vi "h.DETECTION.GetAllChannelDetectionSettingIds.vi"(8 "error in":errorcluster, 11 "Connection ID":refnum<k5>) -> (0 "error out":errorcluster, 2 "Detection Settings IDs":u8[](array[numeric]), 3 "Connection ID out":refnum<k5>)   [LabVIEW 2016, in "h.Library.lvlib"]
uses:
  h.Library.lvlib
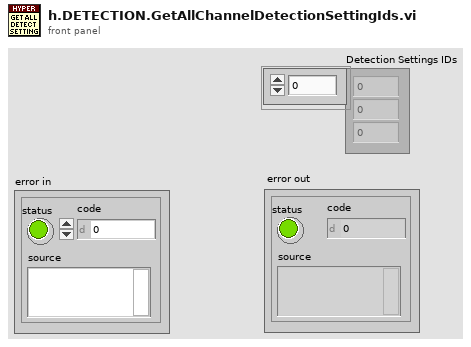
[diagram p1: front panel]
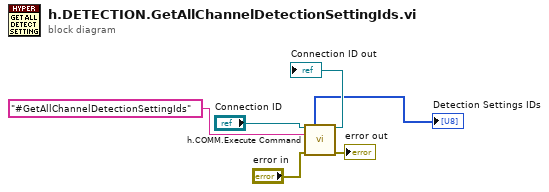
[diagram p0: block diagram]
diagram:
  n1 = call "h.COMM.Execute Command.vi"("Connection ID"="Connection ID", "Command"="#GetAllChannelDetectionSettingIds", "error in"="error in") -> ("Content"=→"Detection Settings IDs":u8[], "Connection ID out"=→"Connection ID out":refnum<k5>, "error out"=→"error out":errorcluster)  [unwired: 5 in, 5 out]
